vi "MAP.vi"(7 "Cmd":enum16{"Init", "Run"}(ring), 8 "error in (no error)":errorcluster, 10 "SLAM In":T1) -> (0 "error out":errorcluster, 2 "SLAM Out":T1, 3 "Landmark Array":cluster{dbl[], dbl[]}, 5 "Robot Position":cluster{dbl[], dbl[]})   [LabVIEW 2009]
uses:
  Controls/SLAM.ctl
  <vilib>/Analysis/Matrix/Datatypes/RealMatrix.ctl
  <vilib>/Analysis/Matrix/NI_Matrix.lvlib
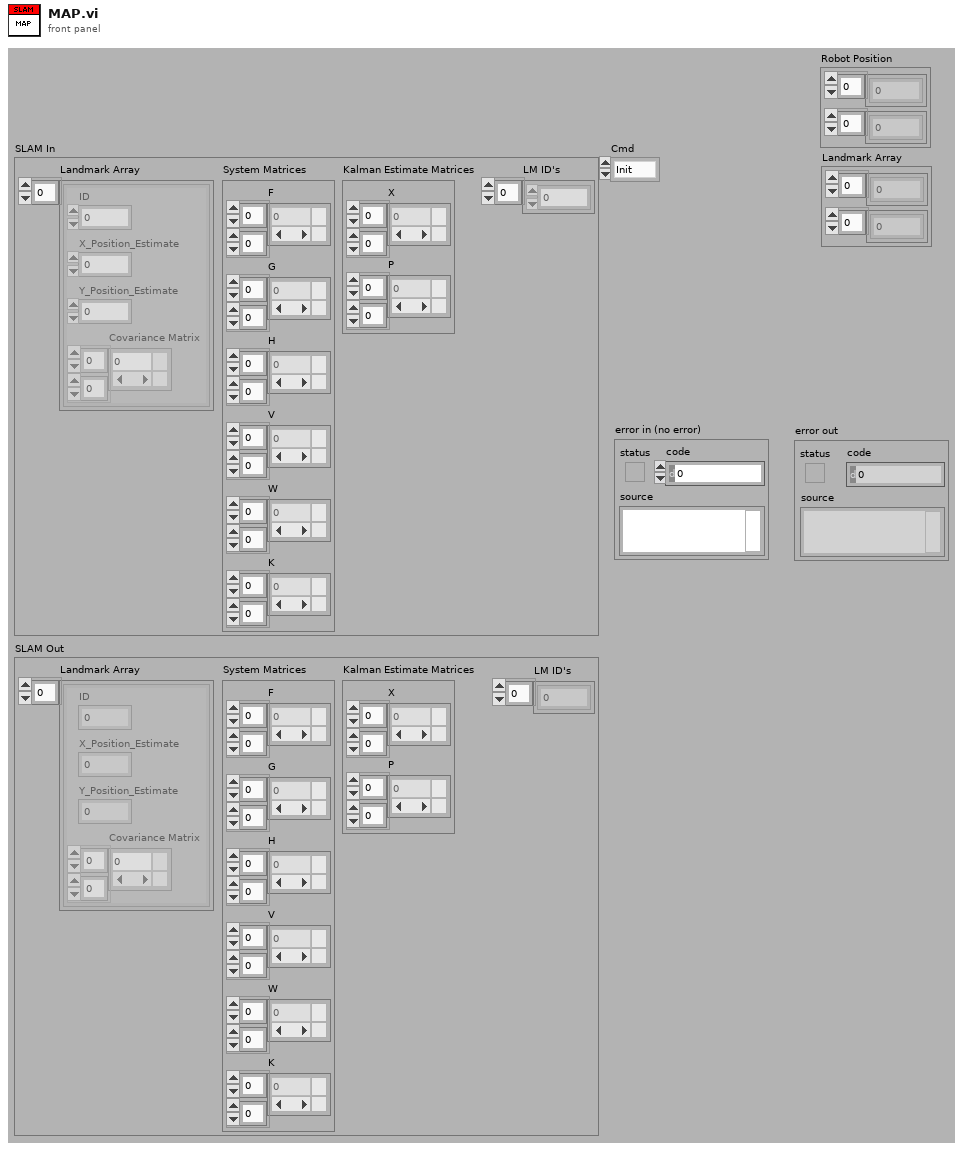
[diagram p1: front panel]
types:
  T1 = typedef "SLAM.ctl" = cluster{"Landmark Array":cluster{"ID":dbl, "X_Position_Estimate":dbl, "Y_Position_Estimate":dbl, "Covariance Matrix":T2}[], "System Matrices":cluster{"F":T2, "G":T2, "H":T2, "V":T2, "W":T2, "K":T2}, "Kalman Estimate Matrices":cluster{"X":T2, "P":T2}, "LM ID's":dbl[]}
  T2 = typedef "NI_Matrix.lvlib/RealMatrix.ctl" = dbl[][]
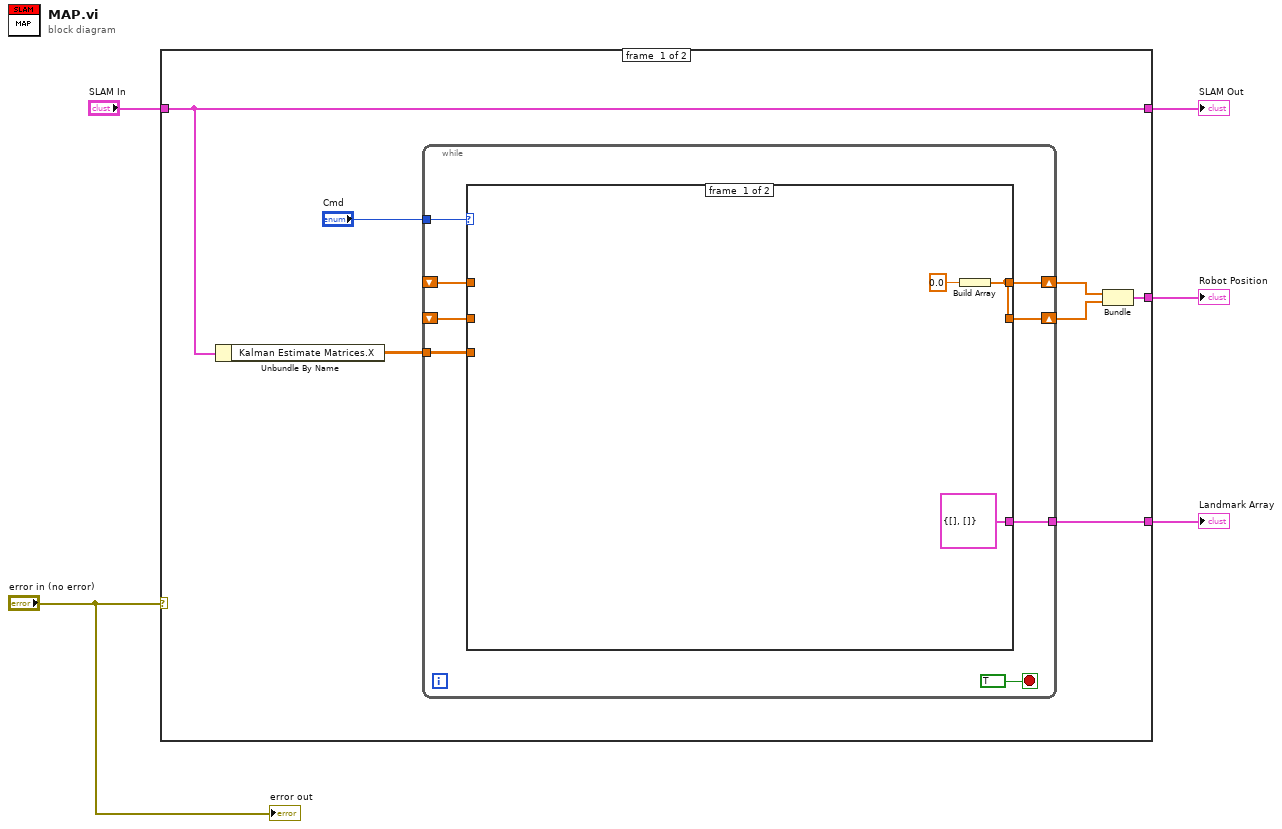
[diagram p0: block diagram]
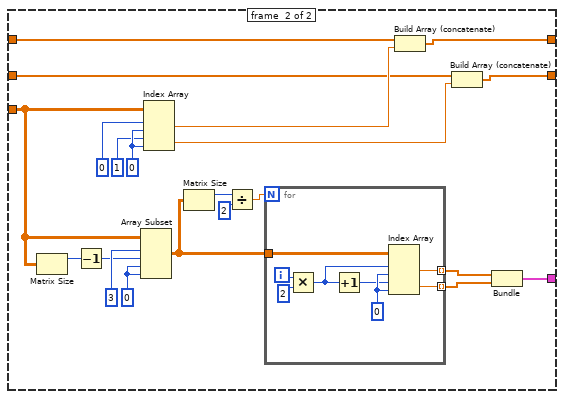
[diagram p2: hidden frame]
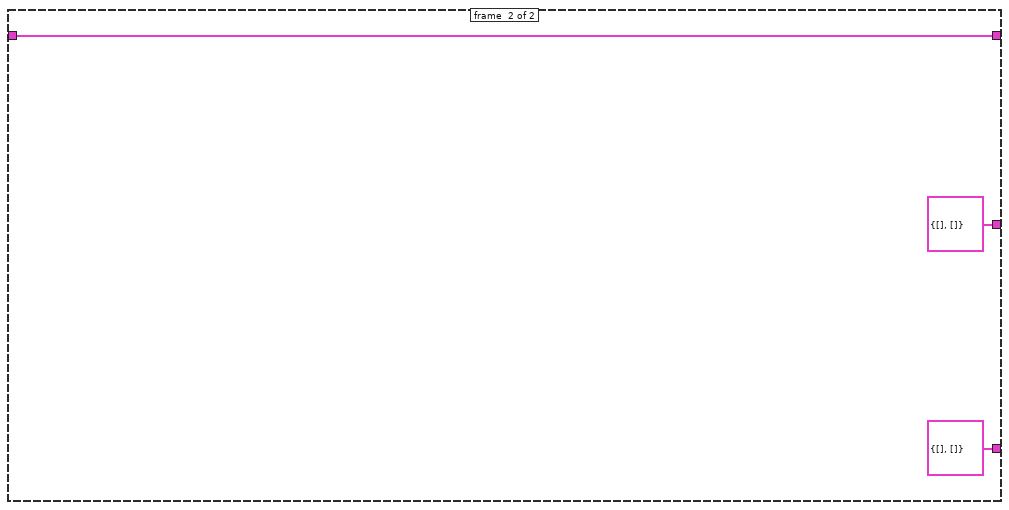
[diagram p3: hidden frame]
diagram:
  n1 = case shown="No Error" "error in (no error)" {
    tunnel: "SLAM In" -> [w10 w55]
    tunnel: [w10 w55] -> w4
    tunnel: [w9 cluster{dbl[], dbl[]} {[], []}] -> w2
    tunnel: [w6 cluster{dbl[], dbl[]} {[], []}] -> w1
    frame #0 {
      n2 = Unbundle By Name(w10) -> ("Kalman Estimate Matrices.X"=w12:T2)
      n3 = while {
        tunnel: w12 -> [w17]
        shift-right: [w15] -> w7
        shift-left: _ -> [w18]
        tunnel: "Cmd" -> [w19]
        shift-right: [w16] -> w8
        shift-left: _ -> [w14]
        tunnel: [w13] -> w6
        stop <- TRUE stop-if-true
        n4 = case shown="\"Run\"" w19 {
          tunnel: w18 -> [_ w38]
          tunnel: w17 -> [_ w33]
          tunnel: [w22 w39] -> w16
          tunnel: [w22 w36] -> w15
          tunnel: w14 -> [_ w41]
          tunnel: [cluster{dbl[], dbl[]} {[], []} w24] -> w13
          frame #0 {
            n5 = Build Array(0.0) -> (w22:dbl[])
          }
          frame #1 {
            w35 = 0 ("index (col)")
            w44 = 0 ("index (col)")
            n6 = Matrix Size(0:w33) -> (1:w32:i32)  [unwired: 1 out]
            n7 = Decrement(x=w32) -> (x-1=w31:i32)
            n8 = Array Subset(array=w33, index (row)=3 ("row 1"), length (row)=w31, index (col)=w35, length (col)=w35) -> (w30:T2)
            n9 = Index Array(array=w33, index (row) #1=0 ("index (col)"), index (col) #1=w44, index (row) #2=1 ("index (col)"), index (col) #2=w44) -> (element #1=w40:dbl, element #2=w37:dbl)
            n10 = Matrix Size(0:w30) -> (1:w29:i32)  [unwired: 1 out]
            n11 = Divide(x=w29, y=2) -> (x/y=w27:dbl)
            n12 = for {
              N: w27 -> [_]
              tunnel: w30 -> [w51]
              tunnel: [w46] -> w26 mode=indexing
              tunnel: [w45] -> w25 mode=indexing
              i -> [w50]
              w52 = 0 ("index (col)")
              n13 = Multiply(x=w50, y=2) -> (x*y=w48:i32)
              n14 = Increment(x=w48) -> (x+1=w47:i32)
              n15 = Index Array(array=w51, index (row) #1=w48, index (col) #1=w52, index (row) #2=w47, index (col) #2=w52) -> (element #1=w46:dbl, element #2=w45:dbl)
            }
            n16 = Build Array (concatenate)(w41, w40) -> (w39:dbl[])
            n17 = Build Array (concatenate)(w38, w37) -> (w36:dbl[])
            n18 = Bundle(w26, w25) -> (w24:cluster{dbl[], dbl[]})  [unwired: 1 in]
          }
        }
      }
      n19 = Bundle(w8, w7) -> (w9:cluster{dbl[], dbl[]})  [unwired: 1 in]
    }
    frame #1 {
    }
  }
  "SLAM Out" <- w4
  "Robot Position" <- w2
  "Landmark Array" <- w1
  "error out" <- "error in (no error)"
